vi "Read Discrete Inputs.vi"(8 "error in (no error)":errorcluster, 9 "number of inputs":u16, 10 "starting address":u16, 11 "device data model in":refnum<class "Device Data Model.lvclass">) -> (0 "error out":errorcluster, 2 "data":bool[](array[boolean]), 3 "device data model out":refnum<class "Device Data Model.lvclass">)   [LabVIEW 2018, in "SubVIs.lvlib" / "Device Data Model.lvclass"]
doc: "Reads N discrete inputs from the data model starting at address M."
uses:
  Device Data Model.lvclass
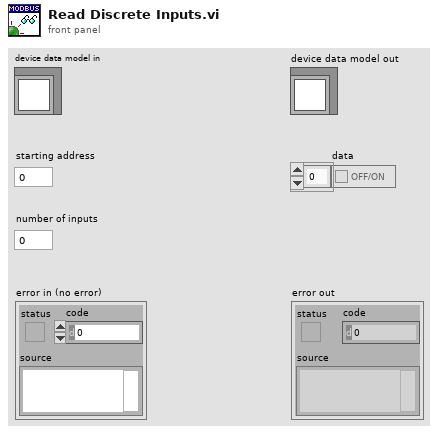
[diagram p1: front panel]
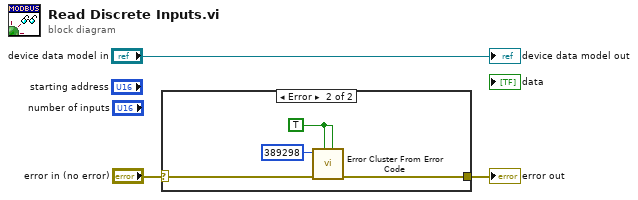
[diagram p0: block diagram]
diagram:
  n1 = case shown="Error" "error in (no error)" {
    selector: "error in (no error)" -> [w4 w8]
    tunnel: [w4 w7] -> w1
    frame No Error {
    }
    frame Error {
      w5 = TRUE ("show call chain? (False)")
      n2 = call "Error Cluster From Error Code.vi"("is warning? (False)"=w5, "show call chain? (False)"=w5, "error in (no error)"=w8, "error code (0)"=389298) -> ("error out"=w7:errorcluster)  [unwired: 5 in]
    }
  }
  "error out" <- w1
  "device data model out" <- "device data model in"
